vi "Page_Exclusions_ReadShared.vi"(8 "error in (no error)":errorcluster, 10 "ctlReferences":T1, 11 "AB_Build in":refnum<class "AB_Build.lvclass">) -> (0 "error out":errorcluster, 3 "AB_Build out":refnum<class "AB_Build.lvclass">)   [LabVIEW 2020, in "AB_Build.lvclass"]
uses:
  <vilib>/AppBuilder/AB_Classes/Build/AB_Build.lvclass
  <resource>/Framework/Providers/Builds/AppBuilder/AB_UI_Page_Exclusions_References.ctl
  <vilib>/AppBuilder/AB_Classes/Build/AB_Build.lvclass/AB_Build.ctl
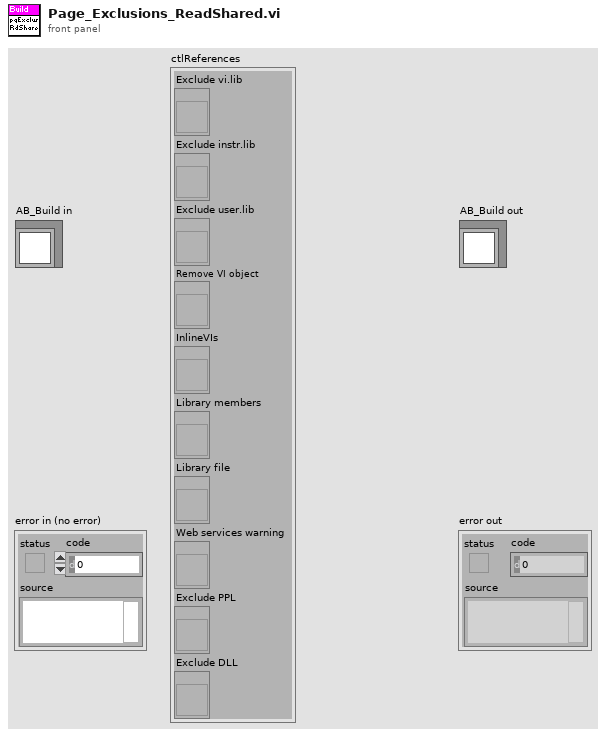
[diagram p1: front panel]
types:
  T1 = typedef "AB_UI_Page_Exclusions_References.ctl" = cluster{"Exclude vi.lib":refnum<vi>, "Exclude instr.lib":refnum<vi>, "Exclude user.lib":refnum<vi>, "Remove VI object":refnum<vi>, "InlineVIs":refnum<vi>, "Library members":refnum<vi>, "Library file":refnum<vi>, "Web services warning":refnum<vi>, "Exclude PPL":refnum<vi>, "Exclude DLL":refnum<vi>}
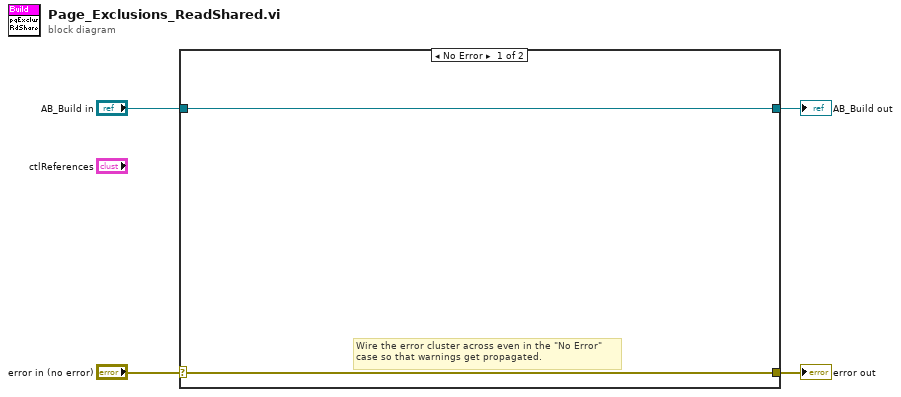
[diagram p0: block diagram]
diagram:
  n1 = case shown="No Error" "error in (no error)" {
    selector: "error in (no error)" -> [w5 w8]
    tunnel: [w5 w8] -> w3
    tunnel: [w6 w7] -> w1
    tunnel: "AB_Build in" -> [w6 w7]
    frame No Error {
      # "Wire the error cluster across even in the \"No Error\"\ncase so that warnings get propagated."
    }
    frame Error {
    }
  }
  "error out" <- w3
  "AB_Build out" <- w1
